vi "Local_pathplanning_박범근(10.28).vi"() -> ()   [LabVIEW 2018]
uses:
  <vilib>/Utility/file.llb/Read Delimited Spreadsheet (DBL).vi
  <vilib>/Analysis/6fits.llb/1D B-Spline Fit.vi
  <vilib>/Analysis/NI_AALPro.lvlib
panel:
  out "카운트":i32
  out "시작":i32
  out "장애물 번호":i32
  out "XY 그래프":cluster{dbl[], dbl[]}(graph)
  in  "반지름 r":dbl(slide) scale=0.0..7.0
  out "충돌가능성(0에 가까우면 충돌)":dbl
  out "충돌위험":bool
  in  "입력 변수 4":dbl
  in  "입력 변수 3":dbl
  in  "입력 변수 2":dbl
  in  "입력 변수":dbl
  in  "장애물 위치":dbl[][](array[numeric])
  out "X 중심점":dbl
  out "Y 중심점":dbl
  in  "정지":bool
  in  "RDDF 불러오기":path
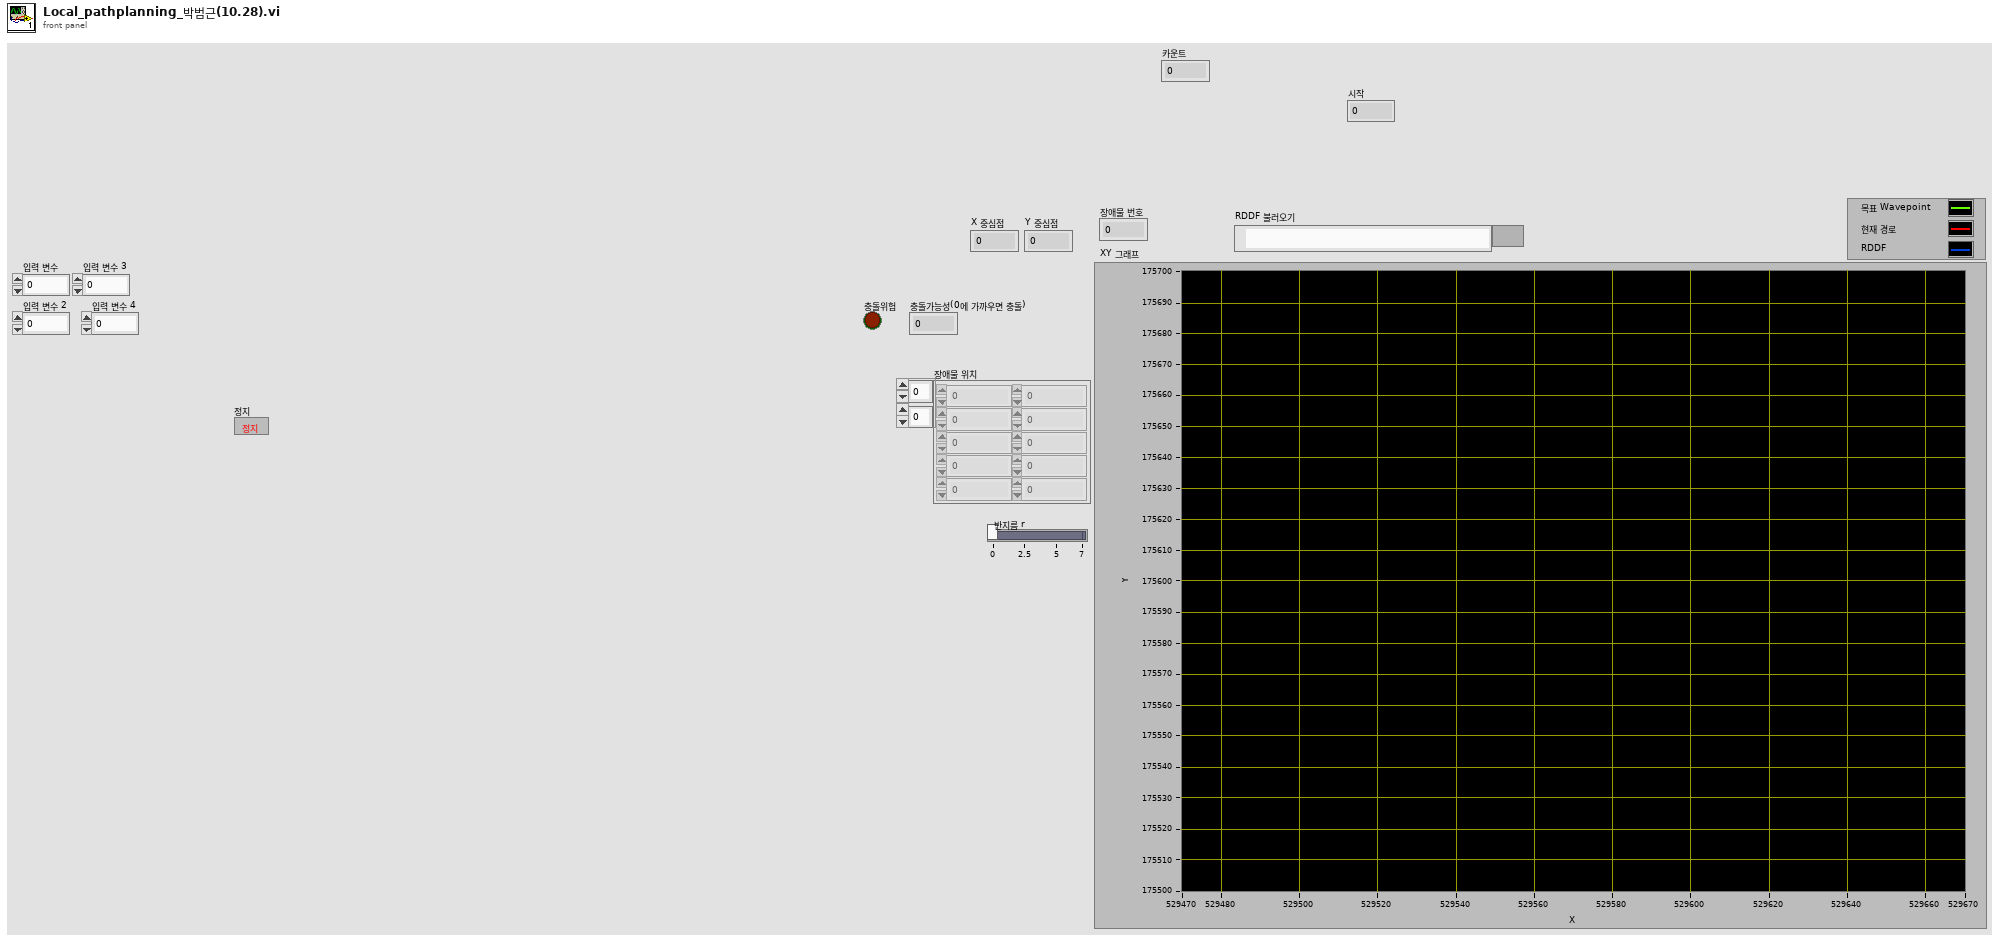
[diagram p1: front panel]
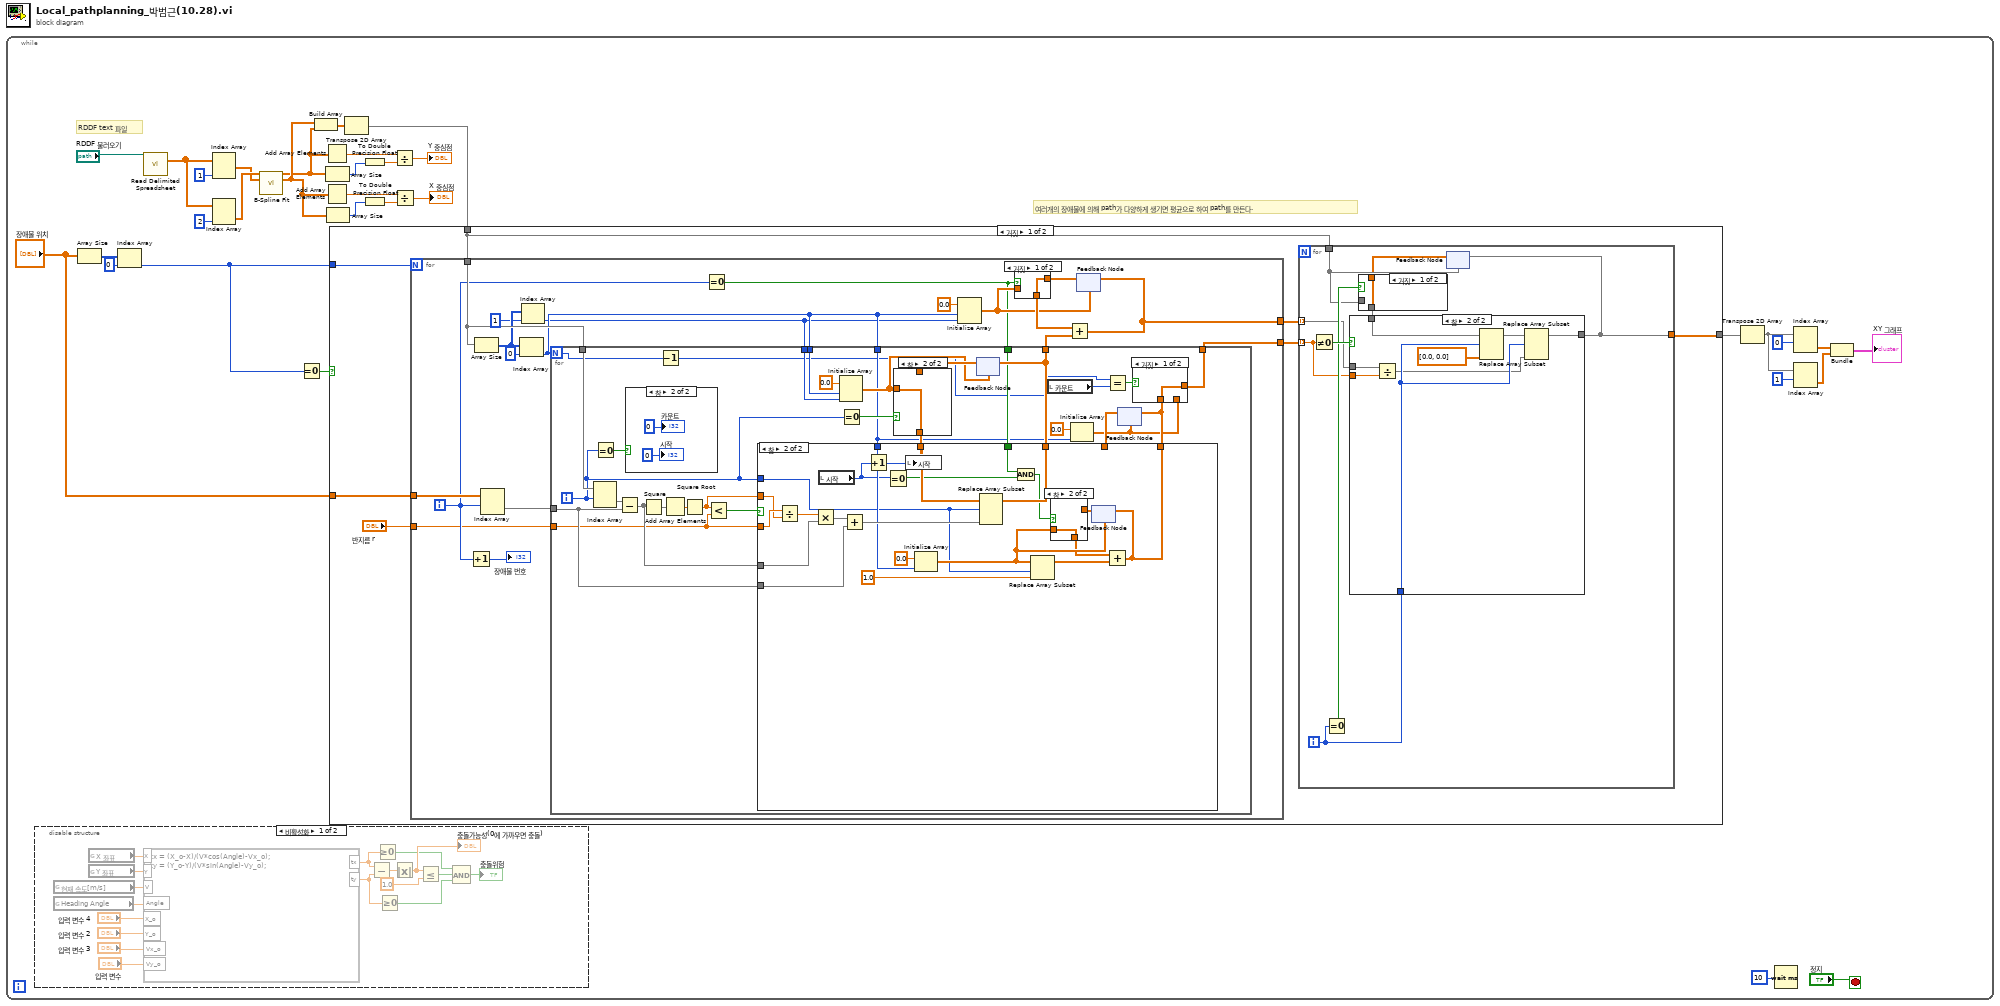
[diagram p0: block diagram]
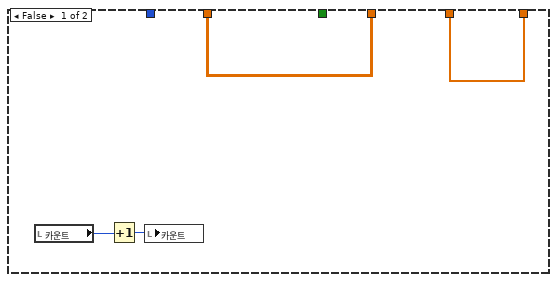
[diagram p9: hidden frame]
diagram:
  n1 = while {
    stop <- "정지" stop-if-true
    # "여러개의 장애물에 의해 path가 다양하게 생기면 평균으로 하여 path를 만든다."
    # "RDDF text 파일"
    n2 = disable-structure shown="비활성화" {
      frame Disabled {
        n3 = global read "글로벌 (10.16).vi" "현재 속도[m/s]"() -> (w47:dbl)
        n4 = global read "글로벌 (10.16).vi" "Heading Angle"() -> (w46:dbl)
        n5 = global read "글로벌 (10.16).vi" "X 좌표"() -> (w49:dbl)
        n6 = global read "글로벌 (10.16).vi" "Y 좌표"() -> (w48:dbl)
        n7 = formula code="tx = (X_o-X)/(V*cos(Angle)-Vx_o);\nty = (Y_o-Y)/(V*sin(Angle)-Vy_o);"("X"=w49, "Y"=w48, "V"=w47, "Angle"=w46, "X_o"="입력 변수 4", "Y_o"="입력 변수 2", "Vx_o"="입력 변수 3", "Vy_o"="입력 변수") -> ("tx"=w38:dbl, "ty"=w37:dbl)
        n8 = Subtract(x=w38, y=w37) -> (x-y=w41:dbl)
        n9 = Greater Or Equal To 0?(x=w38) -> (x >= 0?=w36:bool)
        n10 = Greater Or Equal To 0?(x=w37) -> (x >= 0?=w34:bool)
        n11 = Absolute Value(x=w41) -> (abs(x)=w40:dbl)
        "충돌가능성(0에 가까우면 충돌)" <- w40
        n12 = Less Or Equal?(x=w40, y=1.0) -> (x <= y?=w35:bool)
        n13 = Compound Arithmetic op=AND ("복합 연산")(w36, w35, w34) -> (→"충돌위험":bool)
      }
      frame Enabled {
      }
    }
    n14 = Array Size(array="장애물 위치") -> (size(s)=w14:i32[])
    n15 = Index Array(array=w14, index=0 ("인덱스")) -> (element=w6:i32)
    n16 = call-poly <vilib>:"Read Delimited Spreadsheet.vi"("file path (dialog if empty)"="RDDF 불러오기") -> ("all rows"=w30:dbl[][])  [unwired: 9 in, 5 out]
    n17 = Index Array(array=w30, index (col)=1 ("비활성화된 인덱스 (열)")) -> (element=w27:dbl[])  [unwired: 1 in]
    n18 = Index Array(array=w30, index (col)=2 ("비활성화된 인덱스 (열)")) -> (element=w28:dbl[])  [unwired: 1 in]
    n19 = call-poly <vilib>:"B-Spline Fit.vi"("Y"=w28, "X"=w27) -> ("Best BSpline Fit Y"=w16:dbl[], "Best BSpline Fit X"=w17:dbl[])  [unwired: 10 in, 2 out]
    n20 = Equal To 0?(x=w6) -> (x = 0?=w4:bool)
    n21 = Build Array(w17, w16) -> (w15:dbl[][])
    n22 = Add Array Elements(numeric array=w16) -> (sum=w25:dbl)
    n23 = Array Size(array=w16) -> (size(s)=w23:i32)
    n24 = Add Array Elements(numeric array=w17) -> (sum=w21:dbl)
    n25 = Array Size(array=w17) -> (size(s)=w20:i32)
    n26 = Transpose 2D Array(2D array=w15) -> (transposed array=w5:dbl[][])
    n27 = case shown="거짓" w4 {
      tunnel: "장애물 위치" -> [w56 _]
      tunnel: [w51 w163] -> w3
      tunnel: w6 -> [w55 _]
      tunnel: w5 -> [w52 w163]
      frame False {
        n28 = for {
          N: w55 -> [_]
          tunnel: w56 -> [w95]
          tunnel: w52 -> [w92]
          tunnel: [w81] -> w53
          tunnel: [w80] -> w54
          tunnel: "반지름 r" -> [w77]
          i -> [w79]
          n29 = Increment(x=w79) -> (x+1=→"장애물 번호":i32)
          n30 = Array Size(array=w92) -> (size(s)=w90:i32[])
          n31 = Index Array(array=w95, index (row)=w79) -> (element=w93:dbl[])  [unwired: 1 in]
          n32 = Index Array(array=w90, index=0 ("인덱스")) -> (element=w83:i32)
          n33 = Index Array(array=w90, index=1 ("인덱스")) -> (element=w82:i32)
          n34 = Equal To 0?(x=w79) -> (x = 0?=w84:bool)
          n35 = for {
            N: w83 -> [w103]
            tunnel: w93 -> [w120]
            tunnel: w92 -> [w126]
            tunnel: [w119] -> w91
            tunnel: w83 -> [w108]
            tunnel: w84 -> [w118]
            tunnel: w83 -> [w112]
            tunnel: w82 -> [w111]
            tunnel: [w100] -> w80
            tunnel: w77 -> [w107]
            i -> [w105]
            n36 = Index Array(array=w126, index (row)=w105) -> (element=w127:dbl[])  [unwired: 1 in]
            n37 = Equal To 0?(x=w105) -> (x = 0?=w106:bool)
            n38 = Subtract(x=w127, y=w120) -> (x-y=w121:dbl[])
            n39 = case shown="참" w106 {
              frame False {
              }
              frame True {
                "시작" <- 0 ("숫자형 2")
                "카운트" <- 0 ("카운트")
              }
            }
            n40 = Square(x=w121) -> (x^2=w125:dbl[])
            n41 = Decrement(x=w103) -> (x-1=w102:i32)
            n42 = Add Array Elements(numeric array=w125) -> (sum=w124:dbl)
            n43 = Square Root(x=w124) -> (sqrt(x)=w122:dbl)
            n44 = Less?(x=w122, y=w107) -> (x < y?=w123:bool)
            n45 = Initialize Array(0.0 ("원소"), w112, w111) -> (w113:dbl[][])
            n46 = Equal To 0?(x=w105) -> (x = 0?=w116:bool)
            n47 = feedback #1(w113) -> (w114:dbl[][])
            n48 = case shown="참" w116 {
              tunnel: w113 -> [_ w133]
              tunnel: [w132 w133] -> w115
              tunnel: w114 -> [w132 _]
              frame False {
              }
              frame True {
              }
            }
            n49 = local read "카운트"() -> (w104:i32)
            n50 = Initialize Array(0.0 ("원소"), w108) -> (w99:dbl[])
            n51 = Equal?(x=w102, y=w104) -> (x = y?=w98:bool)
            n52 = feedback #2(w99) -> (w110:dbl[])
            n53 = case shown="참" w123 {
              tunnel: w122 -> [_ w159]
              tunnel: w107 -> [_ w160]
              tunnel: w121 -> [_ w157]
              tunnel: w120 -> [_ w155]
              tunnel: w115 -> [w137 w153]
              tunnel: [w137 w152] -> w119
              tunnel: w108 -> [_ w150]
              tunnel: w118 -> [_ w141]
              tunnel: [w136 w142] -> w101
              tunnel: w110 -> [w136 _]
              tunnel: w105 -> [_ w140]
              frame False {
                n54 = local read "카운트"() -> (w135:i32)
                n55 = Increment(x=w135) -> (x+1=w134:i32)
                n56 = local write "카운트"(w134) -> ()
              }
              frame True {
                n57 = Divide(x=w160, y=w159) -> (x/y=w158:dbl)
                n58 = Multiply(x=w158, y=w157) -> (x*y=w156:dbl[])
                n59 = local read "시작"() -> (w138:i32)
                n60 = Add(x=w156, y=w155) -> (x+y=w154:dbl[])
                n61 = Increment(x=w138) -> (x+1=w139:i32)
                n62 = Equal To 0?(x=w138) -> (x = 0?=w143:bool)
                n63 = local write "시작"(w139) -> ()
                n64 = Initialize Array(0.0 ("원소"), w150) -> (w147:dbl[])
                n65 = Replace Array Subset(array=w153, new element=w154, index (row)=w140) -> (w152:dbl[][])  [unwired: 1 in]
                n66 = And(x=w141, y=w143) -> (x .and. y?=w144:bool)
                n67 = Replace Array Subset(array=w147, new element=1.0 ("새 원소/부분배열"), index=w140) -> (w148:dbl[])
                n68 = feedback #3(w147) -> (w145:dbl[])
                n69 = case shown="참" w144 {
                  tunnel: w147 -> [_ w162]
                  tunnel: [w161 w162] -> w146
                  tunnel: w145 -> [w161 _]
                  frame False {
                  }
                  frame True {
                  }
                }
                n70 = Add(x=w146, y=w148) -> (x+y=w142:dbl[])
                n71 = feedback-in #3(w142) -> ()
              }
            }
            n72 = feedback-in #1(w119) -> ()
            n73 = feedback-in #2(w101) -> ()
            n74 = case shown="거짓" w98 {
              tunnel: w101 -> [w128 _]
              tunnel: [w128 w129] -> w100
              tunnel: w99 -> [_ w129]
              frame False {
              }
              frame True {
              }
            }
          }
          n75 = Initialize Array(0.0 ("원소"), w83, w82) -> (w85:dbl[][])
          n76 = feedback #4(w85) -> (w86:dbl[][])
          n77 = case shown="거짓" w84 {
            tunnel: [w96 w97] -> w87
            tunnel: w86 -> [w96 _]
            tunnel: w85 -> [_ w97]
            frame False {
            }
            frame True {
            }
          }
          n78 = Add(x=w87, y=w91) -> (x+y=w81:dbl[][])
          n79 = feedback-in #4(w81) -> ()
        }
        n80 = for {
          tunnel: w54 -> [w58] mode=indexing
          tunnel: w53 -> [w59] mode=indexing
          tunnel: w52 -> [w62]
          tunnel: [w57] -> w51
          i -> [w64]
          n81 = Not Equal To 0?(x=w58) -> (x != 0?=w65:bool)
          n82 = Equal To 0?(x=w64) -> (x = 0?=w63:bool)
          n83 = feedback #5(w62) -> (w60:dbl[][])
          n84 = case shown="거짓" w63 {
            tunnel: w62 -> [_ w67]
            tunnel: [w66 w67] -> w61
            tunnel: w60 -> [w66 _]
            frame False {
            }
            frame True {
            }
          }
          n85 = case shown="참" w65 {
            tunnel: w64 -> [_ w73]
            tunnel: [w68 w69] -> w57
            tunnel: w61 -> [w68 w75]
            tunnel: w59 -> [_ w71]
            tunnel: w58 -> [_ w72]
            frame False {
            }
            frame True {
              n86 = Divide(x=w71, y=w72) -> (x/y=w70:dbl[])
              n87 = Replace Array Subset(array=w75, new element=dbl[] [0.0, 0.0] ("새 원소/부분배열"), index (row)=w73) -> (w74:dbl[][])  [unwired: 1 in]
              n88 = Replace Array Subset(array=w74, new element=w70, index (row)=w73) -> (w69:dbl[][])  [unwired: 1 in]
            }
          }
          n89 = feedback-in #5(w57) -> ()
        }
      }
      frame True {
      }
    }
    n90 = To Double Precision Float(number=w23) -> (double precision float=w24:dbl)
    n91 = To Double Precision Float(number=w20) -> (double precision float=w22:dbl)
    n92 = Divide(x=w25, y=w24) -> (x/y=→"Y 중심점":dbl)
    n93 = Divide(x=w21, y=w22) -> (x/y=→"X 중심점":dbl)
    n94 = Transpose 2D Array(2D array=w3) -> (transposed array=w10:dbl[][])
    n95 = Wait (ms)(milliseconds to wait=u32 10 ("대기 시간 (ms)")) -> ()  [unwired: 1 out]
    n96 = Index Array(array=w10, index (row)=0 ("비활성화된 인덱스 (열)")) -> (element=w9:dbl[])  [unwired: 1 in]
    n97 = Index Array(array=w10, index (row)=1 ("비활성화된 인덱스 (열)")) -> (element=w8:dbl[])  [unwired: 1 in]
    n98 = Bundle(w9, w8) -> (→"XY 그래프":cluster{dbl[], dbl[]})  [unwired: 1 in]
  }
